vi "Aquisicao_Dados_V.vi"() -> ()   [LabVIEW 2019]
uses:
  <vilib>/Utility/error.llb/DialogType.ctl
  <vilib>/Platform/TimedLoop/XDataNode/timing_clust.ctl
  <vilib>/Platform/TimedLoop/XDataNode/nitl_modes.ctl
  <vilib>/Platform/TimedLoop/XDataNode/wakeup.ctl
  <vilib>/DAQmx/write.llb/DAQmx Write (Analog 1D DBL NChan 1Samp).vi
  <vilib>/DAQmx/read.llb/DAQmx Read (Analog 1D DBL NChan 1Samp).vi
  <vilib>/DAQmx/create/channels.llb/DAQmx Create Channel (AI-Voltage-Basic).vi
  <vilib>/DAQmx/configure/timing.llb/DAQmx Timing (Sample Clock).vi
  <vilib>/DAQmx/create/channels.llb/DAQmx Create Channel (AO-Voltage-Basic).vi
  <vilib>/DAQmx/miscellaneous.llb/DAQmx Fill In Error Info.vi
  <vilib>/platform/TimedLoop/XDataNode/XDataNode.xnode
  <vilib>/Platform/TimedLoop/XDataNode/XDNodeRunTimeDep.lvlib
panel:
  in  "Vinsp":bool
  in  "Vexp":bool
  in  "Frequência respiratória (rpm)":dbl=6.0
  in  "Pressão de referencia [cmH2O]":dbl(slide) scale=0.0..200.0
  in  "?":bool
  in  "Salvar Dados? 3":bool
  out "Pressão no pulmão e Referência":dbl[][](graph)
  out "Segundos":u32
  # "Passo a passo:\n\n1 - Executar o VI;\n2 - Decidir se deseja salvar ou não os dados, caso deseje, pressione o botão \"Salvar dados\";\n3 - Decidir se deseja controlar o sistema em malha aberta ou fechada, caso deseje malha fechada, pressione o botão \"Malha Fechada\";\n3.1 - Em malha fechada, aplique os ganhos do controlador PID na janela PID Gains. Ajuste a referência no botão de deslizamneto. \n        Caso seja necessário, resete o integrador pelo botão \"Resetar PID\";\n3.2 - Em malha aberta, selecione o valor da tensão a ser aplicada na válvula prporcional (-10 a 10 V)\n4 - Ao final, pressione o botão \"STOP\"\n5 - Se desejar visualizar os dados, os mesmo foram salvos em um arquivo .tdms na pasta XXXX, e o nome dele segue o seguinte fomrato \n      \"Daodos_Ano_Mês_Dia_Hora_Segundo\". Para visualizar, utilize o programa SuperViewer."
  # "Controle"
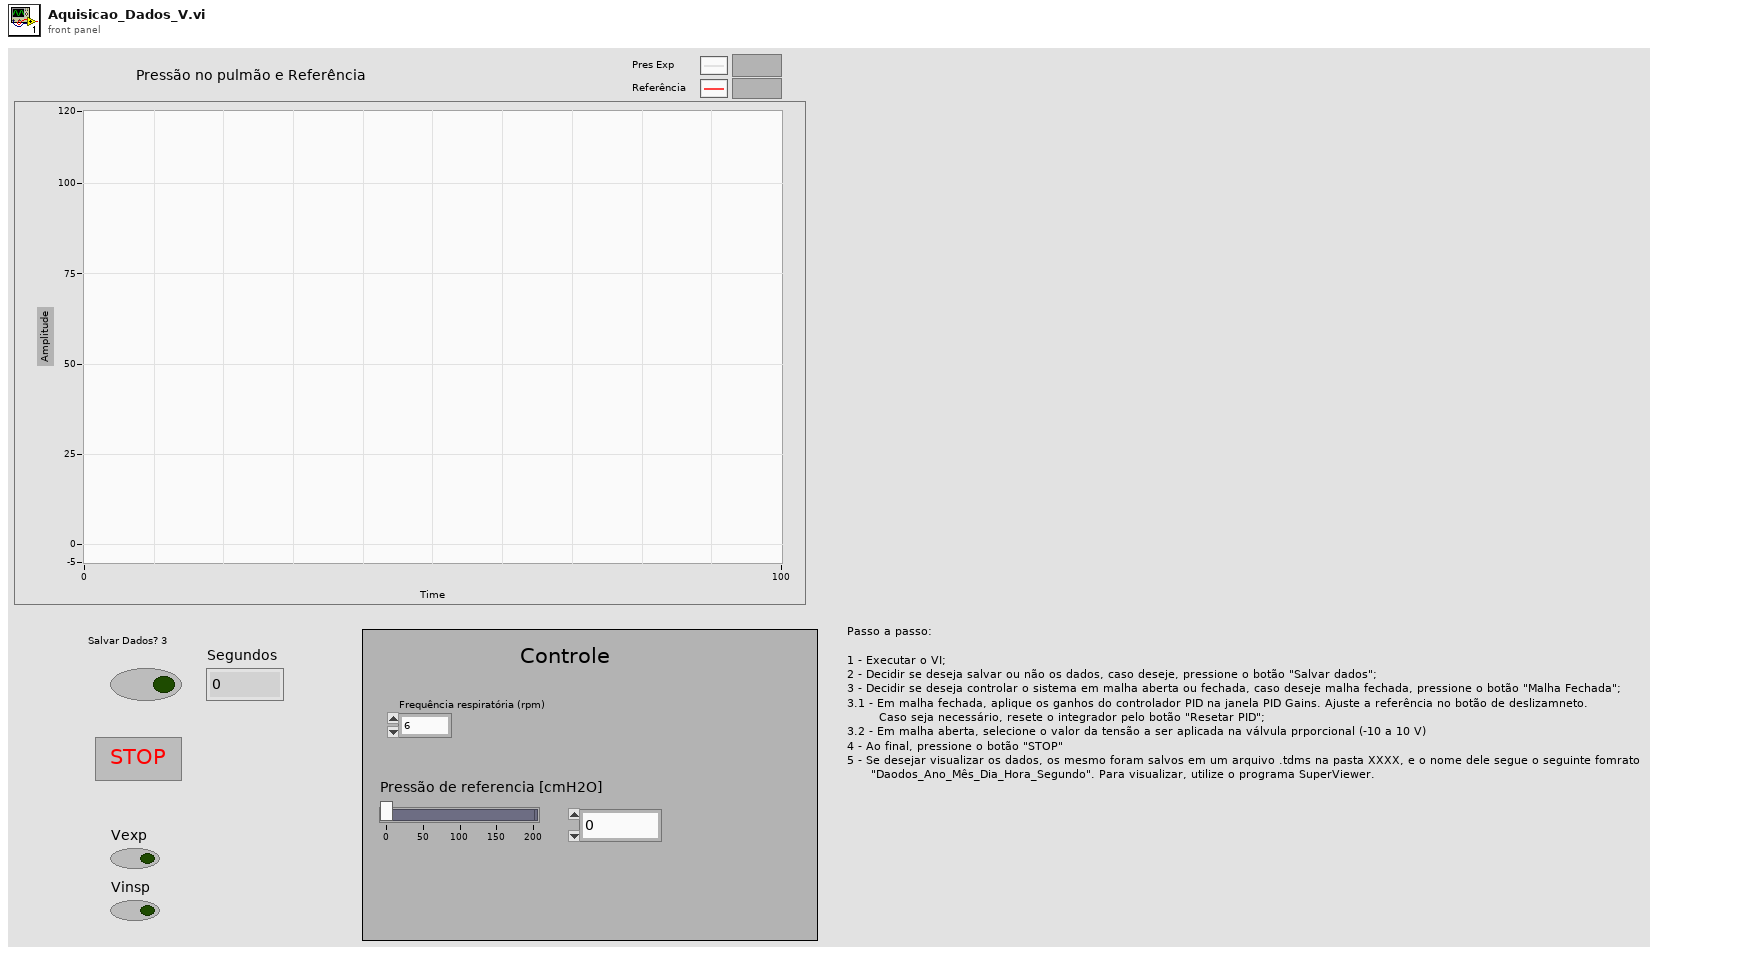
[diagram p1: front panel]
types:
  T1 = enum16{"open", "open or create", "create or replace", "create", "open (read-only)"}
  T2 = typedef "DialogType.ctl" = u16
  T3 = typedef "XDNodeRunTimeDep.lvlib/timing_clust.ctl" = cluster{"Expected End [f-1]":u64, "Actual End [f-1]":u64, "Finished Late? [f-1]":bool, "Expected End [i-1]":u64, "Actual End [i-1]":u64, "Finished Late? [i-1]":bool, "Expected Start [i]":u64, "Actual Start [i]":u64, "Expected Start [f]":u64, "Actual Start [f]":u64, "Source Name":string, "Structure Name":string, "Period":i64, "Deadline":i64, "Offset":i64, "Start":i64, "Priority":i32, "Timeout":i32, "Mode":T4, "Wakeup Reason":T5, "Error":errorcluster, "Source Type":string, "Secondary Source Type":string, "Global End Time":u64, "Global Start Time":u64, "Frame Duration":u64, "Iteration Duration":u64, "Assigned CPU":i32, "I/O Scan Engine Mode":u32}
  T4 = typedef "XDNodeRunTimeDep.lvlib/nitl_modes.ctl" = enum32{"No Change", "Process missed periods, maintain original phase", "Discard missed periods, maintain original phase", "Process missed periods, ignore original phase", "Discard missed periods, ignore original phase"}
  T5 = typedef "XDNodeRunTimeDep.lvlib/wakeup.ctl" = enum32{"Normal", "Aborted", "Asynchronous wakeup", "Timing source error", "Timed loop error", "Timeout"}
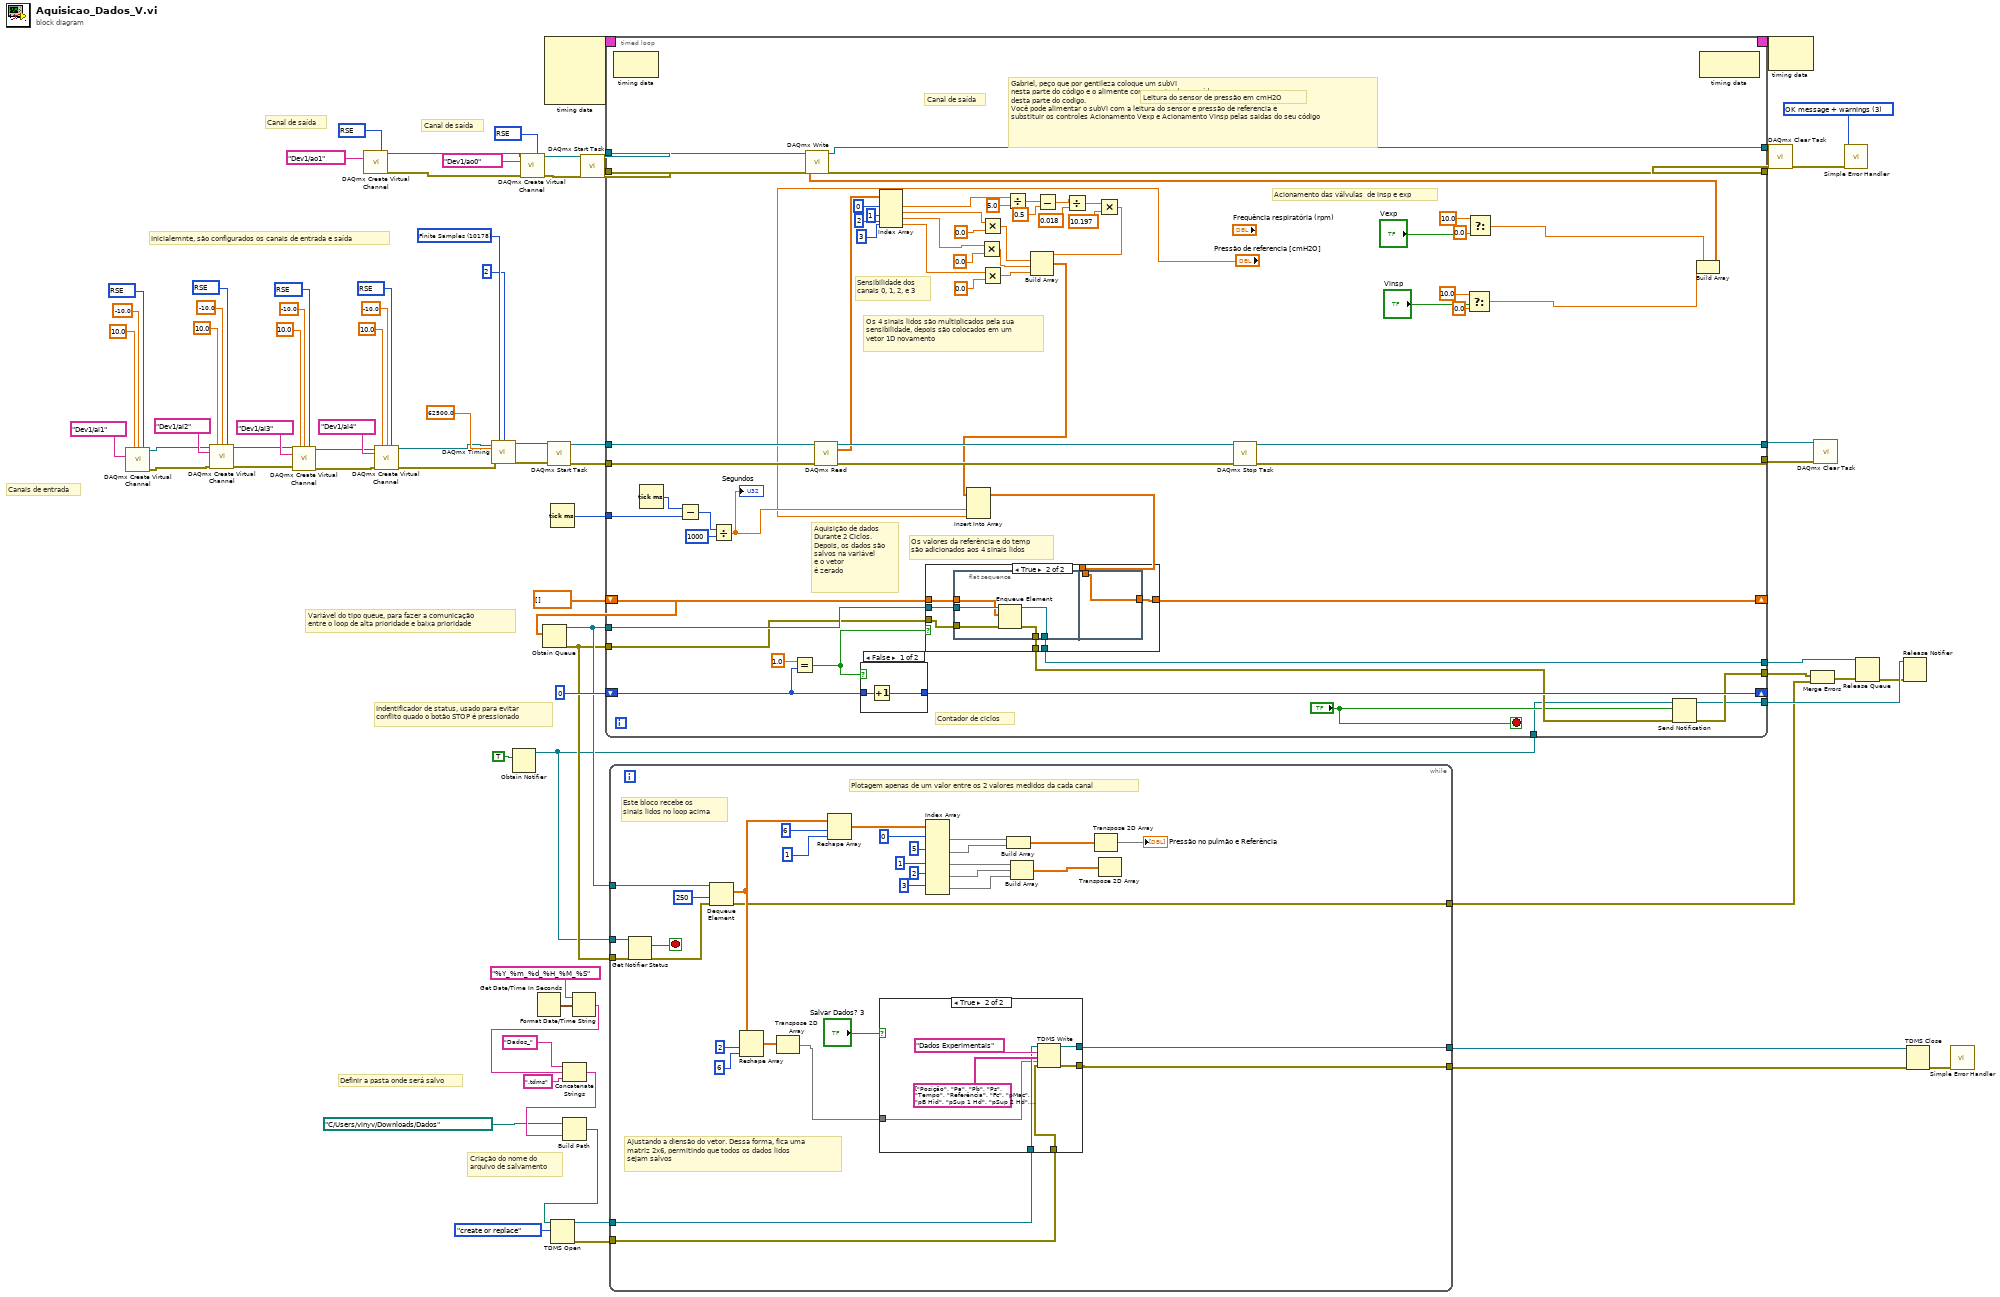
[diagram p0: block diagram]
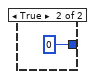
[diagram p2: hidden frame]
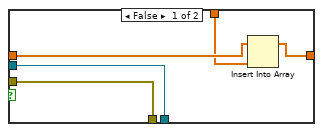
[diagram p3: hidden frame]
diagram:
  w4 = 10083 items=["Default"=-1, "RSE"=10083, "NRSE"=10078, "Differential"=10106, "Pseudodifferential"=12529] ("input terminal configuration")
  w38 = T2 3 items=["no dialog", "OK message", "continue or stop message", "OK message + warnings", "continue/stop + warnings"] ("type of dialog (OK msg:1)")
  w39 = 10083 items=["Default"=-1, "RSE"=10083, "NRSE"=10078, "Differential"=10106, "Pseudodifferential"=12529] ("input terminal configuration")
  w57 = 10083 items=["Default"=-1, "RSE"=10083, "NRSE"=10078, "Differential"=10106, "Pseudodifferential"=12529] ("input terminal configuration")
  w61 = 10083 items=["Default"=-1, "RSE"=10083, "NRSE"=10078, "Differential"=10106, "Pseudodifferential"=12529] ("input terminal configuration")
  w65 = 10083 items=["Default"=-1, "RSE"=10083, "NRSE"=10078, "Differential"=10106, "Pseudodifferential"=12529] ("input terminal configuration")
  w40 = dbl[] []
  w71 = 10178 items=["Finite Samples"=10178, "Continuous Samples"=10123, "Hardware Timed Single Point"=12522] ("sample mode")
  w74 = 10083 items=["Default"=-1, "RSE"=10083, "NRSE"=10078, "Differential"=10106, "Pseudodifferential"=12529] ("input terminal configuration")
  # "Canal de saída"
  # "Definir a pasta onde será salvo"
  # "Indentificador de status, usado para evitar \nconflito quado o botão STOP é pressionado"
  # "Variável do tipo queue, para fazer a comunicação \nentre o loop de alta prioridade e baixa prioridade"
  # "Canais de entrada"
  # "Canal de saída"
  # "Inicialemnte, são configurados os canais de entrada e saída"
  # "Criação do nome do\narquivo de salvamento"
  n1 = call-poly <vilib>:"DAQmx Create Virtual Channel.vi"("maximum value"=10.0, "minimum value"=-10.0, "input terminal configuration"=w57, "physical channels"=tag "Dev1/ai1") -> ("task out"=w53:refnum<k21>, "error out"=w52:errorcluster)  [unwired: 10 in]
  n2 = call-poly <vilib>:"DAQmx Create Virtual Channel.vi"("task in"=w53, "maximum value"=10.0, "minimum value"=-10.0, "input terminal configuration"=w74, "physical channels"=tag "Dev1/ai2", "error in"=w52) -> ("task out"=w51:refnum<k21>, "error out"=w50:errorcluster)  [unwired: 8 in]
  n3 = call-poly <vilib>:"DAQmx Create Virtual Channel.vi"("task in"=w51, "maximum value"=10.0, "minimum value"=-10.0, "input terminal configuration"=w65, "physical channels"=tag "Dev1/ai3", "error in"=w50) -> ("task out"=w49:refnum<k21>, "error out"=w48:errorcluster)  [unwired: 8 in]
  n4 = call-poly <vilib>:"DAQmx Create Virtual Channel.vi"("output terminal configuration"=w4, "physical channels"=tag "Dev1/ao1") -> ("task out"=w2:refnum<k21>, "error out"=w1:errorcluster)  [unwired: 12 in]
  n5 = call-poly <vilib>:"DAQmx Create Virtual Channel.vi"("task in"=w49, "maximum value"=10.0, "minimum value"=-10.0, "input terminal configuration"=w61, "physical channels"=tag "Dev1/ai4", "error in"=w48) -> ("task out"=w47:refnum<k21>, "error out"=w46:errorcluster)  [unwired: 8 in]
  n6 = call-poly <vilib>:"DAQmx Timing.vi"("task/channels in"=w47, "sample mode"=w71, "samples per channel"=2, "rate"=62500.0, "error in"=w46) -> ("task out"=w70:refnum<k21>, "error out"=w69:errorcluster)  [unwired: 9 in]
  n7 = Obtain Notifier(notification data type=TRUE) -> (notifier out=w9:refnum<notifier>)  [unwired: 3 in, 2 out]
  n8 = call-poly <vilib>:"DAQmx Create Virtual Channel.vi"("task in"=w2, "output terminal configuration"=w39, "physical channels"=tag "Dev1/ao0", "error in"=w1) -> ("task out"=w35:refnum<k21>, "error out"=w34:errorcluster)  [unwired: 10 in]
  n9 = Get Date/Time In Seconds() -> (seconds since 1Jan1904=w24:timestamp)
  n10 = Obtain Queue(element data type=w40) -> (queue out=w28:refnum<queue>, error out=w11:errorcluster)  [unwired: 4 in, 1 out]
  n11 = node-c288() -> (w76:T3)  [unwired: 4 in]
  n12 = call <vilib>:"DAQmx Start Task.vi"("task/channels in"=w70, "error in"=w69) -> ("task out"=w45:refnum<k21>, "error out"=w44:errorcluster)  [unwired: 12 in]
  n13 = Tick Count (ms)() -> (millisecond timer value=w29:u32)
  n14 = Format Date/Time String(time format string (%c)="%Y_%m_%d_%H_%M_%S", seconds (now)=w24) -> (date/time string=w25:string)  [unwired: 1 in]
  n15 = Concatenate Strings("Dados_" ("name or relative path"), w25, ".tdms" ("string")) -> (w26:string)
  n16 = Build Path(base path=path "C:/Users/vinyv/Downloads/Dados", name or relative path=w26) -> (appended path=w19:path)
  n17 = TDMS Open(10:T1."create or replace" ("operation (0:open)"), 11:w19) -> (0:w17:errorcluster, 3:w18:refnum<k34>)  [unwired: 5 in]
  n18 = call <vilib>:"DAQmx Start Task.vi"("task/channels in"=w35, "error in"=w34) -> ("task out"=w33:refnum<k21>, "error out"=w32:errorcluster)  [unwired: 12 in]
  n19 = timed-loop {
    timing: w76 -> [_]
    timing-out: [_] -> w75
    tunnel: w45 -> [w140]
    tunnel: w44 -> [w139]
    tunnel: [w120] -> w43
    tunnel: [w119] -> w42
    shift-right: [w137] -> _
    shift-left: 0 -> [w136]
    shift-right: [w117] -> _
    shift-left: w40 -> [w134]
    tunnel: w28 -> [w133]
    tunnel: w11 -> [w132]
    tunnel: [w131] -> w13
    tunnel: [w99] -> w6
    tunnel: w33 -> [w130]
    tunnel: w32 -> [w129]
    tunnel: [w128] -> w31
    tunnel: [w127] -> w30
    tunnel: w29 -> [w125]
    tunnel: [w97] -> w12
    tunnel: w9 -> [w96]
    stop <- "?" stop-if-true
    # "Gabriel, peço que por gentileza coloque um subVI \nnesta parte do código e o alimente com as entradas e saídas \ndesta parte do codigo. \nVocê pode alimentar o subVI com a leitura do sensor e pressão de referencia e \nsubstituir os controles Acionamento Vexp e Acionamento Vinsp pelas saidas do seu código"
    # "Acionamento das válvulas  de insp e exp"
    # "Leitura do sensor de pressão em cmH2O"
    # "Os valores da referência e do temp \nsão adicionados aos 4 sinais lidos"
    # "Os 4 sinais lidos são multiplicados pela sua\nsensibilidade, depois são colocados em um \nvetor 1D novamento"
    # "Canal de saída"
    # "Sensibilidade dos \ncanais 0, 1, 2, e 3"
    # "Contador de ciclos"
    # "Aquisição de dados\nDurante 2 Ciclos. \nDepois, os dados são\nsalvos na variável\ne o vetor\né zerado"
    n20 = node-c288() -> ()  [unwired: 1 in, 1 out]
    n21 = Tick Count (ms)() -> (millisecond timer value=w126:u32)
    n22 = Subtract(x=w126, y=w125) -> (x-y=w124:u32)
    n23 = Divide(x=w124, y=u32 1000) -> (x/y=w118:dbl)
    "Segundos" <- w118
    n24 = Equal?(x=1.0, y=w136) -> (x = y?=w135:bool)
    n25 = call-poly <vilib>:"DAQmx Read.vi"("task/channels in"=w140, "error in"=w139) -> ("task out"=w121:refnum<k21>, "data"=w115:dbl[], "error out"=w122:errorcluster)  [unwired: 11 in]
    n26 = case shown="False" w135 {
      tunnel: [w142 0] -> w137
      tunnel: w136 -> [w141 _]
      frame False {
        n27 = Increment(x=w141) -> (x+1=w142:i32)
      }
      frame True {
      }
    }
    n28 = Index Array(array=w115, index #1=0 ("index"), index #2=1 ("index"), index #3=2 ("index"), index #4=3 ("index")) -> (element #1=w94:dbl, element #2=w107:dbl, element #3=w106:dbl, element #4=w105:dbl)
    n29 = Multiply(x=w106, y=0.0) -> (x*y=w103:dbl)
    n30 = Multiply(x=w107, y=0.0) -> (x*y=w104:dbl)
    n31 = Multiply(x=w105, y=0.0) -> (x*y=w102:dbl)
    n32 = Divide(x=w94, y=5.0 ("x")) -> (x/y=w92:dbl)
    n33 = Subtract(x=w92, y=0.5) -> (x-y=w90:dbl)
    n34 = Divide(x=w90, y=0.018) -> (x/y=w88:dbl)
    n35 = Multiply(x=w88, y=10.197) -> (x*y=w86:dbl)
    n36 = Build Array(w86, w104, w103, w102) -> (w101:dbl[])
    n37 = Insert Into Array(array=w101, new element #1=w118, new element #2="Pressão de referencia [cmH2O]") -> (w116:dbl[])  [unwired: 1 in]
    n38 = case shown="True" w135 {
      tunnel: [w148 w155] -> w117
      tunnel: w134 -> [w147 w150]
      tunnel: w133 -> [w146 w154]
      tunnel: w132 -> [w145 w153]
      tunnel: [w146 w152] -> w131
      tunnel: [w145 w151] -> w100
      tunnel: w116 -> [w144 w149]
      frame False {
        n39 = Insert Into Array(array=w147, new element=w144) -> (w148:dbl[])  [unwired: 1 in]
      }
      frame True {
        n40 = flat-sequence {
          tunnel: w154 -> [w160]
          tunnel: w153 -> [w159]
          tunnel: [w158] -> w152
          tunnel: [w157] -> w151
          tunnel: w150 -> [w156]
          tunnel: [w161] -> w155
          tunnel: w149 -> [w161]
          frame #0 {
            n41 = Enqueue Element(queue=w160, element=w156, error in (no error)=w159) -> (queue out=w158:refnum<queue>, error out=w157:errorcluster)  [unwired: 1 in, 1 out]
          }
          frame #1 {
          }
        }
      }
    }
    n42 = call <vilib>:"DAQmx Stop Task.vi"("task/channels in"=w121, "error in"=w122) -> ("task out"=w120:refnum<k21>, "error out"=w119:errorcluster)  [unwired: 12 in]
    n43 = Select(t=10.0, s="Vinsp", f=0.0) -> (s? t:f=w83:dbl)
    n44 = Select(t=10.0, s="Vexp", f=0.0) -> (s? t:f=w84:dbl)
    n45 = Send Notification(notification="?", notifier=w96, error in (no error)=w100) -> (notifier out=w97:refnum<notifier>, error out=w99:errorcluster)
    n46 = Build Array(w84, w83) -> (w95:dbl[])
    n47 = call-poly <vilib>:"DAQmx Write.vi"("task/channels in"=w130, "data"=w95, "error in"=w129) -> ("task out"=w128:refnum<k21>, "error out"=w127:errorcluster)  [unwired: 10 in, 1 out]
    n48 = node-c288() -> ()  [unwired: 1 in, 1 out]
  }
  n49 = while {
    tunnel: w28 -> [w185]
    tunnel: w18 -> [w183]
    tunnel: w17 -> [w182]
    tunnel: [w181] -> w15
    tunnel: [w180] -> w14
    tunnel: w9 -> [w169]
    tunnel: w11 -> [w168]
    tunnel: [w165] -> w7
    stop <- w166 stop-if-true
    # "Este bloco recebe os \nsinais lidos no loop acima"
    # "Ajustando a diensão do vetor. Dessa forma, fica uma \nmatriz 2x6, permitindo que todos os dados lidos \nsejam salvos"
    # "Plotagem apenas de um valor entre os 2 valores medidos da cada canal"
    n50 = Get Notifier Status(notifier=w169, error in (no error)=w168) -> (current notification=w166:bool, error out=w167:errorcluster)  [unwired: 3 out]
    n51 = Dequeue Element(queue=w185, timeout in ms (-1)=250, error in (no error)=w167) -> (element=w176:dbl[], error out=w165:errorcluster)  [unwired: 2 out]
    n52 = Reshape Array(w176, 2 ("dimension size"), 6 ("dimension size")) -> (w178:dbl[][])
    n53 = Transpose 2D Array(2D array=w178) -> (transposed array=w177:dbl[][])
    n54 = Reshape Array(w176, 6 ("dimension size"), 1 ("dimension size")) -> (w189:dbl[][])
    n55 = case shown="True" "Salvar Dados? 3" {
      tunnel: w183 -> [w197 w203]
      tunnel: w182 -> [w198 w202]
      tunnel: [w197 w201] -> w181
      tunnel: [w198 w200] -> w180
      tunnel: w177 -> [_ w199]
      frame False {
      }
      frame True {
        n56 = TDMS Write(0:w203, 5:"Dados Experimentais" ("group name in (Untitled)"), 7:string[] ["Posição", "Pa", "Pb", "Ps", "Tempo", "Referência", "Fc", "pMac", "pB Hid", "pSup 1 Hd", "pSup 2 Hd", "pA Pn", "pB Pn", "Enc", "Tempo", "Ta", "Tb", "Ts", "Velocidade"] ("channel name(s) in (Untitled)"), 9:w199, 11:w202) -> (4:w201:refnum<k34>, 15:w200:errorcluster)  [unwired: 1 in, 2 out]
      }
    }
    n57 = Index Array(array=w189, index (row) #1=0 ("index (row)"), index (row) #2=5 ("index (row)"), index (row) #3=1 ("index (row)"), index (row) #4=2 ("index (row)"), index (row) #5=3 ("index (row)")) -> (element #1=w186:dbl[], element #2=w190:dbl[], element #3=w172:dbl[], element #4=w171:dbl[], element #5=w170:dbl[])  [unwired: 5 in]
    n58 = Build Array(w186, w190) -> (w188:dbl[][])
    n59 = Build Array(w172, w171, w170) -> (w175:dbl[][])
    n60 = Transpose 2D Array(2D array=w188) -> (transposed array=→"Pressão no pulmão e Referência":dbl[][])
    n61 = Transpose 2D Array(2D array=w175) -> ()  [unwired: 1 out]
  }
  n62 = node-c288(w75) -> ()  [unwired: 1 out]
  n63 = call <vilib>:"DAQmx Clear Task.vi"("task in"=w31, "error in"=w30) -> ("error out"=w37:errorcluster)  [unwired: 13 in]
  n64 = Merge Errors(w6, w7) -> (w5:errorcluster)
  n65 = call <vilib>:"DAQmx Clear Task.vi"("task in"=w43, "error in"=w42) -> ()  [unwired: 13 in, 1 out]
  n66 = call <vilib>:"Simple Error Handler.vi"("type of dialog (OK msg:1)"=w38, "error in (no error)"=w37) -> ()  [unwired: 3 in, 5 out]
  n67 = Release Queue(queue=w13, error in (no error)=w5) -> (error out=w8:errorcluster)  [unwired: 1 in, 2 out]
  n68 = Release Notifier(notifier=w12, error in (no error)=w8) -> ()  [unwired: 1 in, 3 out]
  n69 = TDMS Close(8:w14, 11:w15) -> (0:w16:errorcluster)  [unwired: 1 out]
  n70 = call <vilib>:"Simple Error Handler.vi"("error in (no error)"=w16) -> ()  [unwired: 4 in, 5 out]
